vi "Parse.vi"(10 "String In":string, 11 "RegEx":string="StatusCode") -> (2 "After String":string, 3 "Content":string)   [LabVIEW 2016, in "Response.lvclass"]
uses:
  Response.lvclass
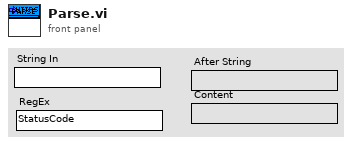
[diagram p1: front panel]
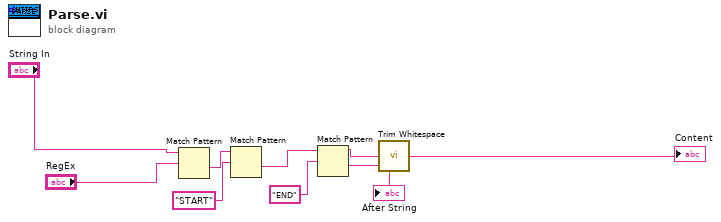
[diagram p0: block diagram]
diagram:
  n1 = Match Pattern(string="String In", regular expression="RegEx") -> (after substring=w4:string)  [unwired: 1 in, 3 out]
  n2 = Match Pattern(string=w4, regular expression="START") -> (after substring=w6:string)  [unwired: 1 in, 3 out]
  n3 = Match Pattern(string=w6, regular expression="END") -> (before substring=w8:string, after substring=→"After String":string)  [unwired: 1 in, 2 out]
  n4 = call <vilib>:"Trim Whitespace.vi"("string"=w8) -> ("trimmed string"=→"Content":string)  [unwired: 1 in]
